vi "test_RS-xxx to GPIB ConvBox Close.vi"(8 "error in (no error)":errorcluster, 11 "TestCase in":refnum<class "Instrument Addon Serial Protocols Unit Tests.lvclass">) -> (0 "error out":errorcluster, 3 "TestCase out":refnum<class "Instrument Addon Serial Protocols Unit Tests.lvclass">)   [LabVIEW 2023, in "Instrument Addon Serial Protocols Unit Tests.lvclass"]
uses:
  Instrument Addon Serial Protocols Unit Tests.lvclass
  <vilib>/addons/_JKI Toolkits/VI Tester/TestCase.llb/TestCase.lvclass
  Listener/ListenerClassControls/Operation.ctl
  Listener/Listener.lvclass
  RS-xxx to GPIB ConvBox/RS-xxx to GPIB ConvBox.lvclass
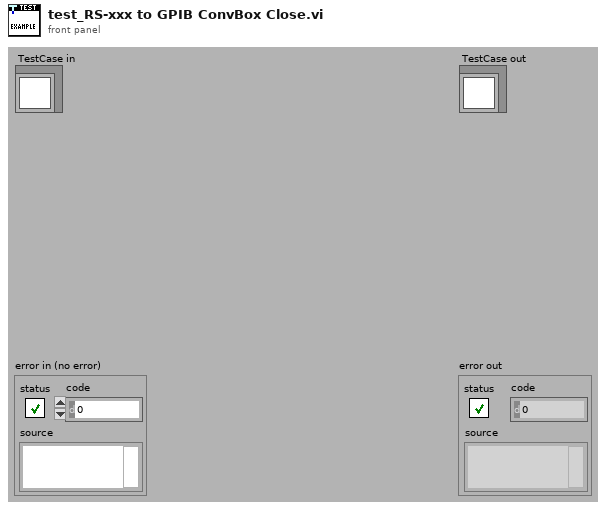
[diagram p1: front panel]
types:
  T1 = typedef "Listener.lvclass/Operation.ctl" = enum16{"Read", "Write"}
  T2 = typedef "Listener.lvclass/RS-xxx To GPIB ConvBox Data Structure.ctl" = cluster{"Data":string, "Command Messages Read":string[], "Address":string, "Data Length":u32}
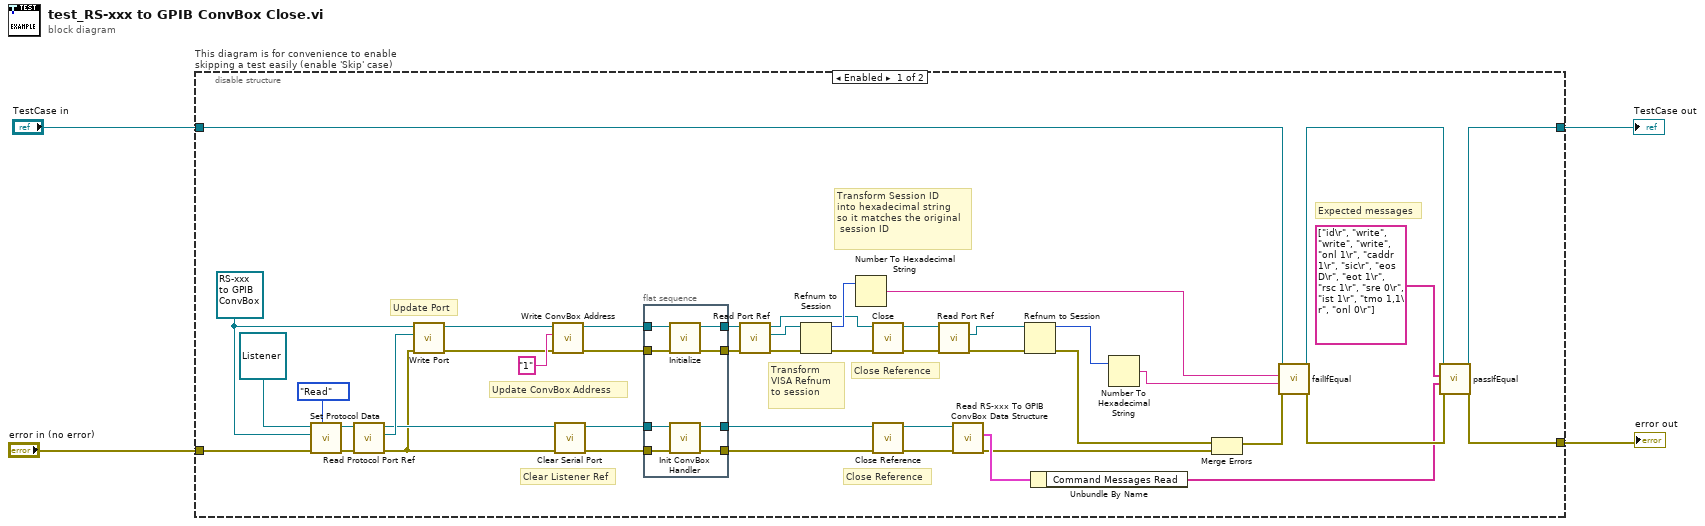
[diagram p0: block diagram]
diagram:
  n1 = disable-structure "This diagram is for convenience to enable skipping a test easily (enable 'Skip' case)" shown="Enabled" {
    disable-tunnel: "TestCase in" -> [w49 w61]
    disable-tunnel: [w9 w59] -> w1
    disable-tunnel: [w11 w60] -> w3
    disable-tunnel: "error in (no error)" -> [w48 w58]
    frame Enabled {
      w37 = refnum<class "RS-xxx to GPIB ConvBox.lvclass"> refnum ("Protocols.lvlib:RS-xxx to GPIB ConvBox.lvclass")
      # "Close Reference"
      # "Close Reference"
      # "Transform Session ID \ninto hexadecimal string\nso it matches the original\n session ID"
      # "Transform \nVISA Refnum \nto session"
      # "Update Port"
      # "Expected messages"
      # "Update ConvBox Address"
      # "Clear Listener Ref"
      n2 = call "Set Protocol Data.vi"("Operation"=Operation."Read", "error in (no error)"=w48, "Protocols.lvlib:Protocol Parent.lvclass"=w37, "Listener In.lvclass"=refnum<class "Listener.lvclass"> refnum ("Listener.lvclass")) -> ("error out"=w41:errorcluster, "Listener Out.lvclass"=w40:refnum<class "Listener.lvclass">)  [unwired: 6 in]
      n3 = call "Read Protocol Port Ref.vi"("error in (no error)"=w41, "Listener in"=w40) -> ("error out"=w34:errorcluster, "Protocol Port Ref"=w36:refnum<visa-resource-name>, "Listener out"=w35:refnum<class "Listener.lvclass">)  [unwired: 7 in]
      n4 = call "Write Port.vi"("error in (no error)"=w34, "Port"=w36, "RS232 to GPIB ConvBox in"=w37) -> ("error out"=w39:errorcluster, "RS232 to GPIB ConvBox out"=w38:refnum<class "RS-xxx to GPIB ConvBox.lvclass">)  [unwired: 7 in]
      n5 = call "Write ConvBox Address.vi"("error in (no error)"=w39, "ConvBox Address"="1", "RS232 to GPIB ConvBox in"=w38) -> ("error out"=w33:errorcluster, "RS232 to GPIB ConvBox out"=w32:refnum<class "RS-xxx to GPIB ConvBox.lvclass">)  [unwired: 7 in]
      n6 = call "Clear Serial Port.vi"("error in (no error)"=w34, "Listener In.lvclass"=w35) -> ("error out"=w44:errorcluster, "Listener out"=w43:refnum<class "Listener.lvclass">)  [unwired: 8 in]
      n7 = flat-sequence {
        tunnel: w44 -> [w57]
        tunnel: w43 -> [w56]
        tunnel: w33 -> [w55]
        tunnel: w32 -> [w54]
        tunnel: [w53] -> w31
        tunnel: [w52] -> w30
        tunnel: [w51] -> w17
        tunnel: [w50] -> w16
        frame #0 {
          n8 = call-dynamic "Initialize.vi"("error in (no error)"=w55, "RS232 to GPIB ConvBox in"=w54) -> ("error out"=w53:errorcluster, "RS232 to GPIB ConvBox out"=w52:refnum<class "RS-xxx to GPIB ConvBox.lvclass">)  [unwired: 8 in]
          n9 = call "Init ConvBox Handler.vi"("error in (no error)"=w57, "Listener in"=w56) -> ("error out"=w51:errorcluster, "Listener out"=w50:refnum<class "Listener.lvclass">)  [unwired: 8 in]
        }
      }
      n10 = call "Read Port Ref.vi"("error in (no error)"=w31, "RS232 to GPIB ConvBox in"=w30) -> ("error out"=w29:errorcluster, "Port Ref"=w27:refnum<visa-resource-name>, "RS232 to GPIB ConvBox out"=w24:refnum<class "RS-xxx to GPIB ConvBox.lvclass">)  [unwired: 7 in]
      n11 = Refnum to Session(4:w29, 7:w27) -> (0:w25:errorcluster, 3:w28:u64)
      n12 = Number To Hexadecimal String(2:w28) -> (0:w26:string)  [unwired: 1 in]
      n13 = call-dynamic "Close.vi"("error in (no error)"=w25, "RS232 to GPIB ConvBox in"=w24) -> ("error out"=w22:errorcluster, "RS232 to GPIB ConvBox out"=w23:refnum<class "RS-xxx to GPIB ConvBox.lvclass">)  [unwired: 8 in]
      n14 = call "Close Reference.vi"("error in (no error)"=w17, "Listener In.lvclass"=w16) -> ("error out"=w13:errorcluster, "Listener out"=w14:refnum<class "Listener.lvclass">)  [unwired: 8 in]
      n15 = call "Read Port Ref.vi"("error in (no error)"=w22, "RS232 to GPIB ConvBox in"=w23) -> ("error out"=w21:errorcluster, "Port Ref"=w20:refnum<visa-resource-name>)  [unwired: 7 in, 1 out]
      n16 = call-dynamic "Read RS-xxx To GPIB ConvBox Data Structure.vi"("error in (no error)"=w13, "Listener in"=w14) -> ("error out"=w7:errorcluster, "RS-xxx To GPIB ConvBox Data Structure"=w8:T2)  [unwired: 7 in, 1 out]
      n17 = Refnum to Session(4:w21, 7:w20) -> (0:w15:errorcluster, 3:w19:u64)
      n18 = Unbundle By Name(w8) -> ("Command Messages Read"=w6:string[])
      n19 = Number To Hexadecimal String(2:w19) -> (0:w18:string)  [unwired: 1 in]
      n20 = Merge Errors(w15, w7) -> (w42:errorcluster)
      n21 = call-dynamic "failIfEqual.vi"("error in (no error)"=w42, "y"=w18, "x"=w26, "TestCase in"=w49) -> ("error out"=w12:errorcluster, "TestCase out"=w10:refnum<class "Instrument Addon Serial Protocols Unit Tests.lvclass">)  [unwired: 6 in]
      n22 = call-dynamic "passIfEqual.vi"("error in (no error)"=w12, "y"=w6, "x"=string[] ["id\r", "write", "write", "write", "onl 1\r", "caddr 1\r", "sic\r", "eos D\r", "eot 1\r", "rsc 1\r", "sre 0\r", "ist 1\r", "tmo 1,1\r", "onl 0\r"] ("Command Messages Read"), "TestCase in"=w10) -> ("error out"=w11:errorcluster, "TestCase out"=w9:refnum<class "Instrument Addon Serial Protocols Unit Tests.lvclass">)  [unwired: 6 in]
    }
    frame Disabled {
      # "skip test result while test is under development"
      n23 = call <vilib>:"skip.vi"("error in (no error)"=w58, "TestCase in"=w61) -> ("error out"=w60:errorcluster, "TestCase out"=w59:refnum<class "Instrument Addon Serial Protocols Unit Tests.lvclass">)  [unwired: 8 in]
    }
  }
  "error out" <- w3
  "TestCase out" <- w1
